vi "Write FPGA Ref.vi"(8 "error in (no error)":errorcluster, 10 "FPGA Ref":refnum<k20>, 11 "FPGA Vaisala in":refnum<class "FPGA Vaisala.lvclass">) -> (0 "error out":errorcluster, 3 "FPGA Vaisala out":refnum<class "FPGA Vaisala.lvclass">)   [LabVIEW 2013, in "FPGA Vaisala.lvclass"]
uses:
  FPGA Vaisala.lvclass
  FPGA Vaisala.lvclass/FPGA Vaisala.ctl
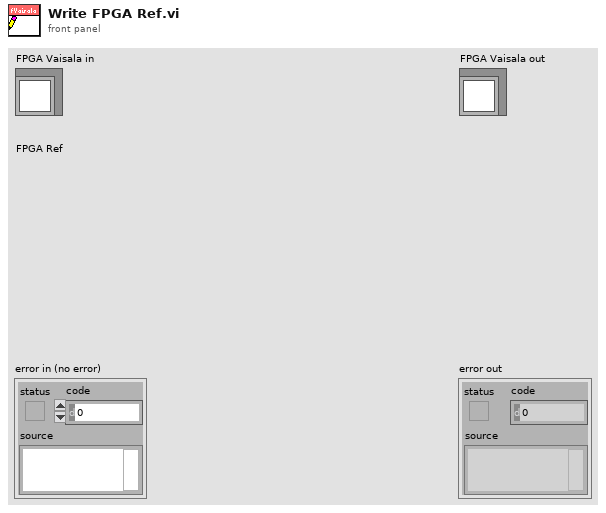
[diagram p1: front panel]
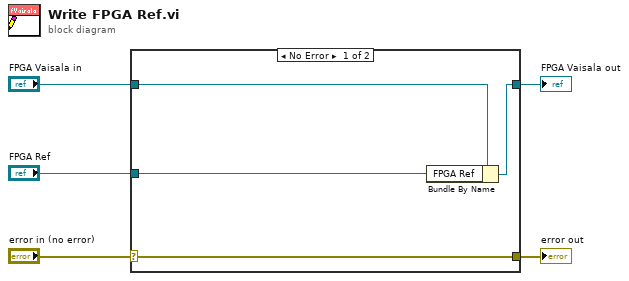
[diagram p0: block diagram]
diagram:
  n1 = case shown="No Error" "error in (no error)" {
    selector: "error in (no error)" -> [w9 w10]
    tunnel: [w9 w10] -> w4
    tunnel: [w7 w11] -> w2
    tunnel: "FPGA Vaisala in" -> [w8 w11]
    tunnel: "FPGA Ref" -> [w6 _]
    frame No Error {
      n2 = Bundle By Name(cluster=w8, "FPGA Ref"=w6) -> (w7:refnum<class "FPGA Vaisala.lvclass">)
    }
    frame Error {
    }
  }
  "error out" <- w4
  "FPGA Vaisala out" <- w2
